vi "Temp to 5K then auto.vi"() -> ()   [LabVIEW 2009, in "Magnet.lvclass"]
uses:
  Magnet.lvclass
panel:
  out "temp":dbl caption="Temperature" format="%#_8g"
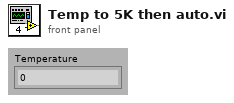
[diagram p1: front panel]
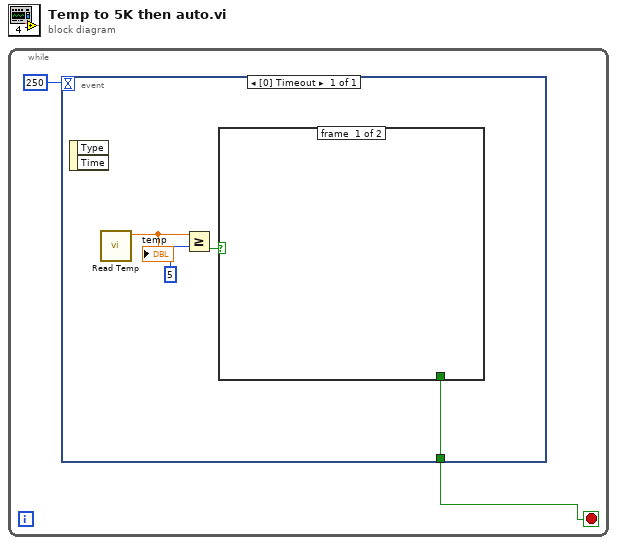
[diagram p0: block diagram]
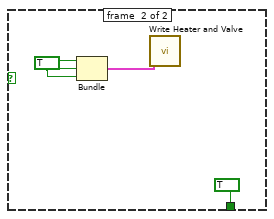
[diagram p2: hidden frame]
diagram:
  n1 = while {
    stop <- w1 stop-if-true
    n2 = event shown="[0] Timeout" {
      selector: _ -> [_]
      dyn-events: _ -> [_]
      timeout: 250 -> [_]
      tunnel: [w3] -> w1
      event [0] Timeout {
        n3 = event-data() -> ()  [unwired: 3 out]
        n4 = call "Read Temp.vi"() -> ("temp"=w6:dbl)  [unwired: 7 out]
        "temp" <- w6
        n5 = Greater Or Equal?(x=w6, y=5) -> (x >= y?=w4:bool)
        n6 = case shown="True" w4 {
          tunnel: [_ TRUE] -> w3
          frame #0 {
          }
          frame #1 {
            w7 = TRUE
            n7 = Bundle(w7, w7, w7) -> (w8:cluster{bool, bool, bool})  [unwired: 1 out]
            n8 = call "Write Heater and Valve.vi"("autoIN"=w8) -> ()  [unwired: 2 in, 9 out]
          }
        }
      }
    }
  }
